vi "Execute.vi"(8 "error in (no error)":errorcluster, 9 "Workspace":T1, 10 "Cluster":T2={"I-O.lvclass"=refnum, "Gantry"=refnum, "Dispenser"="COM1"}, 11 "Pick and Place in":refnum<class "Pick and Place.lvclass">) -> (0 "error out":errorcluster, 2 "Control Out":T2={"I-O.lvclass"=refnum, "Gantry"=refnum, "Dispenser"="COM1"}, 3 "Pick and Place out":refnum<class "Pick and Place.lvclass">)   [LabVIEW 2021, in "Pick and Place.lvclass"]
uses:
  Pick and Place.lvclass
  Controller/Controllers.ctl
  Controller/I-O/I-O.lvclass
  C:/Program Files (x86)/Aerotech/A3200/LabVIEW/2010/Bin/Aerotech.A3200.dll
  Program Files (x86)/Aerotech/A3200/LabVIEW/2010/Bin/Aerotech.A3200.dll
  Workspace/Workspace.ctl
  Pick and Place.lvclass/Pick and Place.ctl
  Controller/Motion/Motion.lvclass
  Controller/Motion/A3200/A3200.lvclass
  Controller/Controller.lvclass
  Workspace/Fixture.lvclass
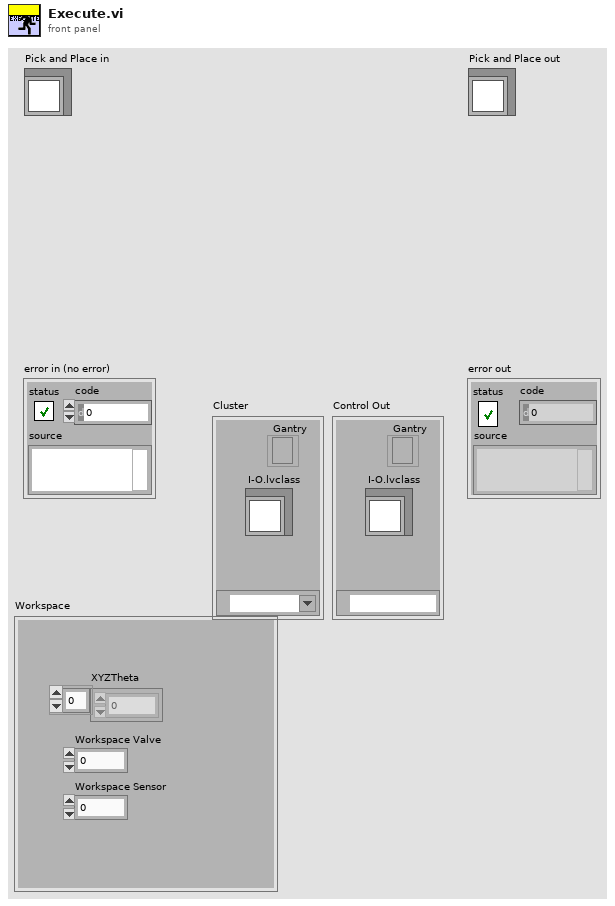
[diagram p1: front panel]
types:
  T1 = typedef "Fixture.lvclass/Workspace.ctl" = cluster{"XYZTheta":dbl[], "Workspace Valve":i32, "Workspace Sensor":i32}
  T2 = typedef "Controller.lvclass/Controllers.ctl" = cluster{"I-O.lvclass":refnum<class "I-O.lvclass">, "Gantry":refnum<k24>, "Dispenser":refnum<visa-resource-name>}
  T3 = typedef "Pick and Place.lvclass/Pick and Place Type.ctl" = enum16{"Primary Pick Up", "Secondary Pick Up", "Put Down All", "Pick Up All", "Put Down Secondary"}
  T4 = typedef "I-O.lvclass/Pin Map.ctl" = cluster{"Region Valves":i32[], "Extra Valves":dbl[][][], "Tool Primary Valve":i32, "Tool Secondary Valve":i32, "Region Sensors":i32[], "Extra Sensors":dbl[][][], "Tool Primary Sensor":dbl, "Tool Secondary Sensor":dbl, "Compression Sensor":dbl, "5V":i32, "Dispenser Sensor":dbl}
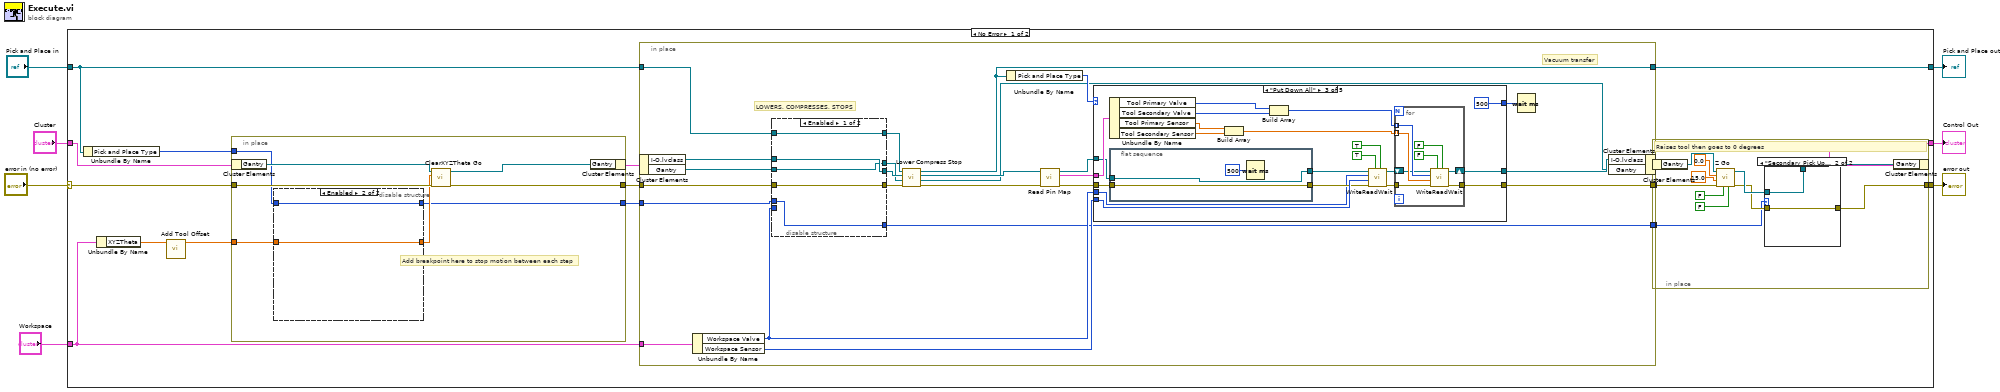
[diagram p0: block diagram]
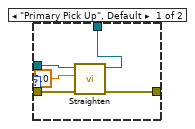
[diagram p2: hidden frame]
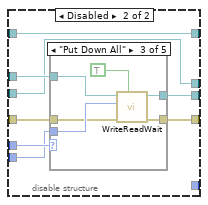
[diagram p3: hidden frame]
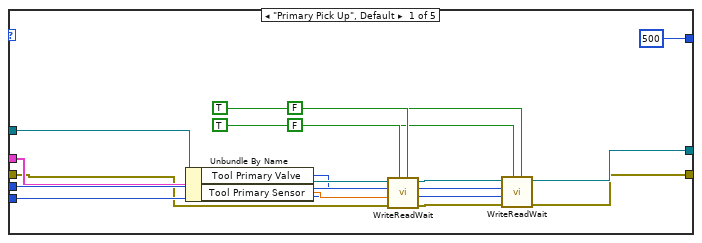
[diagram p8: hidden frame]
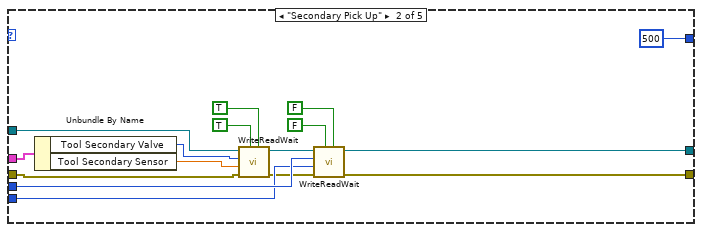
[diagram p9: hidden frame]
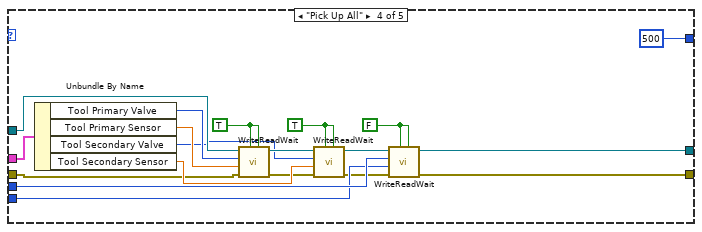
[diagram p10: hidden frame]
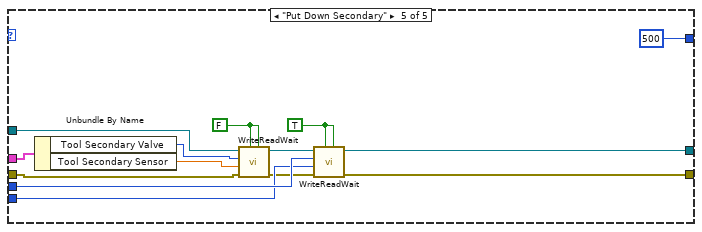
[diagram p11: hidden frame]
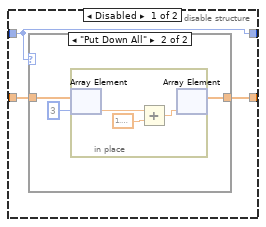
[diagram p12: hidden frame]
diagram:
  n1 = case shown="No Error" "error in (no error)" {
    selector: "error in (no error)" -> [w17 w210]
    tunnel: "Cluster" -> [w21 w211]
    tunnel: "Workspace" -> [w22 _]
    tunnel: [w16 w210] -> w1
    tunnel: [w20 w211] -> w2
    tunnel: "Pick and Place in" -> [w11 w209]
    tunnel: [w19 w209] -> w6
    frame No Error {
      n2 = Unbundle By Name(w11) -> ("Pick and Place Type"=w10:T3)
      n3 = Unbundle By Name(w22) -> ("XYZTheta"=w14:dbl[])
      n4 = call "Add Tool Offset.vi"("XYZTheta"=w14) -> ("Array"=w18:dbl[])  [unwired: 10 in]
      n5 = in-place {
        in-place-border: w18 -> [w191]
        in-place-border: w17 -> [w193]
        in-place-border: [w194] -> w13
        in-place-border: w10 -> [w192]
        in-place-border: [w189] -> w9
        # "Add breakpoint here to stop motion between each step"
        n6 = in-place-cluster #1(w21) -> ("Gantry"=w196:refnum<k24>)
        n7 = disable-structure shown="Enabled" {
          disable-tunnel: w192 -> [w197 w207]
          disable-tunnel: w191 -> [w199 w208]
          disable-tunnel: [w198 w208] -> w190
          disable-tunnel: [w197 w207] -> w189
          frame Disabled {
            n8 = case shown="\"Put Down All\"" w197 {
              tunnel: w199 -> [w200 w203]
              tunnel: [w200 w201] -> w198
              frame "Primary Pick Up", Default {
              }
              frame "Put Down All" {
                n9 = in-place {
                  n10 = in-place-array #2(w203, 3) -> (w206:dbl)
                  n11 = Add(x=w206, y=1.5707963267948966) -> (x+y=w204:dbl)
                  n12 = in-place-array #2(w204) -> (w201:dbl[])  [unwired: 1 out]
                }
              }
            }
          }
          frame Enabled {
          }
        }
        n13 = call "ClearXYZTheta Go.vi"("error in (no error)"=w193, "XYZTheta In"=w190, "Gantry In"=w196) -> ("error out"=w194:errorcluster, "Gantry Out"=w195:refnum<k24>)  [unwired: 6 in, 1 out]
        n14 = in-place-cluster #1("Gantry"=w195) -> (w23:T2)
      }
      n15 = in-place {
        in-place-border: w22 -> [w65]
        in-place-border: w11 -> [w51]
        in-place-border: [w57] -> w19
        in-place-border: w13 -> [w46]
        in-place-border: [w53] -> w12
        in-place-border: w9 -> [w44]
        in-place-border: [w42] -> w8
        # "Vacuum transfer"
        # "LOWERS, COMPRESSES, STOPS"
        n16 = in-place-cluster #3(w23) -> ("I-O.lvclass"=w50:refnum<class "I-O.lvclass">, "Gantry"=w48:refnum<k24>)
        n17 = Unbundle By Name(w65) -> ("Workspace Valve"=w43:i32, "Workspace Sensor"=w63:i32)
        n18 = disable-structure shown="Enabled" {
          disable-tunnel: [w70 w76] -> w52
          disable-tunnel: w51 -> [w70 w76]
          disable-tunnel: w50 -> [w69 w75]
          disable-tunnel: [w69 w74] -> w49
          disable-tunnel: w48 -> [w68 w73]
          disable-tunnel: [w68 w73] -> w47
          disable-tunnel: w46 -> [w67 w72]
          disable-tunnel: [w67 w71] -> w45
          disable-tunnel: w44 -> [w66 w78]
          disable-tunnel: w43 -> [_ w77]
          disable-tunnel: [w66 _] -> w42
          frame Enabled {
          }
          frame Disabled {
            n19 = case shown="\"Put Down All\"" w78 {
              tunnel: w77 -> [_ _ w88 _ _]
              tunnel: w75 -> [w80 w82 w86 w90 w92]
              tunnel: [w80 w82 w85 w90 w92] -> w74
              tunnel: w72 -> [w79 w81 w84 w89 w91]
              tunnel: [w79 w81 w83 w89 w91] -> w71
              frame "Primary Pick Up", Default {
              }
              frame "Secondary Pick Up" {
              }
              frame "Put Down All" {
                n20 = call "WriteReadWait.vi"("Write Value"=TRUE, "error in (no error)"=w84, "Write"=w88, "I-O in"=w86) -> ("error out"=w83:errorcluster, "I-O out"=w85:refnum<class "I-O.lvclass">)  [unwired: 6 in]
              }
              frame "Pick Up All" {
              }
              frame "Put Down Secondary" {
              }
            }
          }
        }
        n21 = call "Lower Compress Stop.vi"("error in (no error)"=w45, "Gantry In"=w47, "I-O.lvclass"=w49, "Pick and Place in"=w52) -> ("error out"=w55:errorcluster, "Gantry Out"=w56:refnum<k24>, "I-O out"=w58:refnum<class "I-O.lvclass">, "Pick and Place Out"=w57:refnum<class "Pick and Place.lvclass">)  [unwired: 4 in]
        n22 = Unbundle By Name(w57) -> ("Pick and Place Type"=w64:T3)
        n23 = call-dynamic "Read Pin Map.vi"("error in (no error)"=w55, "I-O in"=w58) -> ("error out"=w54:errorcluster, "Pin Map 2"=w61:T4, "I-O out"=w60:refnum<class "I-O.lvclass">)  [unwired: 7 in]
        n24 = case shown="\"Put Down All\"" w64 {
          tunnel: w43 -> [w105 w116 w125 w164 w182]
          tunnel: w63 -> [w104 w115 w134 w163 w181]
          tunnel: [w99 w114 w138 w161 w179] -> w59
          tunnel: [u32 500 ("milliseconds to wait") 500 500 u32 500 ("milliseconds to wait") u32 500 ("milliseconds to wait")] -> w62
          tunnel: w60 -> [w98 w113 w130 w173 w187]
          tunnel: w61 -> [w97 w112 w133 w174 w188]
          tunnel: w54 -> [w95 w111 w127 w159 w177]
          tunnel: [w93 w109 w126 w156 w175] -> w53
          frame "Primary Pick Up", Default {
            n25 = Unbundle By Name(w97) -> ("Tool Primary Valve"=w96:i32, "Tool Primary Sensor"=w107:dbl)
            n26 = call "WriteReadWait.vi"("Read Value"=TRUE, "Write Value"=TRUE, "error in (no error)"=w95, "Read"=w107, "Write"=w96, "I-O in"=w98) -> ("error out"=w94:errorcluster, "I-O out"=w106:refnum<class "I-O.lvclass">)  [unwired: 4 in]
            n27 = call "WriteReadWait.vi"("Read Value"=FALSE ("Write Value"), "Write Value"=FALSE ("Read Value"), "error in (no error)"=w94, "Read"=w104, "Write"=w105, "I-O in"=w106) -> ("error out"=w93:errorcluster, "I-O out"=w99:refnum<class "I-O.lvclass">)  [unwired: 4 in]
          }
          frame "Secondary Pick Up" {
            n28 = Unbundle By Name(w112) -> ("Tool Secondary Valve"=w118:i32, "Tool Secondary Sensor"=w117:dbl)
            n29 = call "WriteReadWait.vi"("Read Value"=TRUE, "Write Value"=TRUE, "error in (no error)"=w111, "Read"=w117, "Write"=w118, "I-O in"=w113) -> ("error out"=w110:errorcluster, "I-O out"=w123:refnum<class "I-O.lvclass">)  [unwired: 4 in]
            n30 = call "WriteReadWait.vi"("Read Value"=FALSE ("Write Value"), "Write Value"=FALSE ("Read Value"), "error in (no error)"=w110, "Read"=w115, "Write"=w116, "I-O in"=w123) -> ("error out"=w109:errorcluster, "I-O out"=w114:refnum<class "I-O.lvclass">)  [unwired: 4 in]
          }
          frame "Put Down All" {
            n31 = Unbundle By Name(w133) -> ("Tool Primary Valve"=w139:i32, "Tool Secondary Valve"=w140:i32, "Tool Primary Sensor"=w141:dbl, "Tool Secondary Sensor"=w142:dbl)
            n32 = flat-sequence {
              tunnel: [w146] -> w131
              tunnel: w130 -> [w146]
              tunnel: [w145] -> w128
              tunnel: w127 -> [w145]
              frame #0 {
                # "Delay After Placing"
                n33 = Wait (ms)(milliseconds to wait=u32 500) -> ()  [unwired: 1 out]
              }
            }
            n34 = Build Array(w141, w142) -> (w144:dbl[])
            n35 = Build Array(w139, w140) -> (w143:i32[])
            n36 = call "WriteReadWait.vi"("Read Value"=TRUE, "Write Value"=TRUE, "error in (no error)"=w128, "Read"=w134, "Write"=w125, "I-O in"=w131) -> ("error out"=w129:errorcluster, "I-O out"=w132:refnum<class "I-O.lvclass">)  [unwired: 4 in]
            n37 = for {
              shift-right: [w150] -> w138
              shift-left: w132 -> [w151]
              tunnel: w143 -> [w153] mode=indexing
              tunnel: w144 -> [w152] mode=indexing
              tunnel: w129 -> [w149]
              tunnel: [w148] -> w126
              n38 = call "WriteReadWait.vi"("Read Value"=FALSE ("Write Value"), "Write Value"=FALSE ("Read Value"), "error in (no error)"=w149, "Read"=w152, "Write"=w153, "I-O in"=w151) -> ("error out"=w148:errorcluster, "I-O out"=w150:refnum<class "I-O.lvclass">)  [unwired: 4 in]
            }
          }
          frame "Pick Up All" {
            w162 = FALSE ("Read Value")
            w166 = TRUE ("Write Value")
            w172 = TRUE ("Write Value")
            n39 = Unbundle By Name(w174) -> ("Tool Primary Valve"=w171:i32, "Tool Primary Sensor"=w170:dbl, "Tool Secondary Valve"=w168:i32, "Tool Secondary Sensor"=w167:dbl)
            n40 = call "WriteReadWait.vi"("Read Value"=w172, "Write Value"=w172, "error in (no error)"=w159, "Read"=w170, "Write"=w171, "I-O in"=w173) -> ("error out"=w158:errorcluster, "I-O out"=w169:refnum<class "I-O.lvclass">)  [unwired: 4 in]
            n41 = call "WriteReadWait.vi"("Read Value"=w166, "Write Value"=w166, "error in (no error)"=w158, "Read"=w167, "Write"=w168, "I-O in"=w169) -> ("error out"=w157:errorcluster, "I-O out"=w165:refnum<class "I-O.lvclass">)  [unwired: 4 in]
            n42 = call "WriteReadWait.vi"("Read Value"=w162, "Write Value"=w162, "error in (no error)"=w157, "Read"=w163, "Write"=w164, "I-O in"=w165) -> ("error out"=w156:errorcluster, "I-O out"=w161:refnum<class "I-O.lvclass">)  [unwired: 4 in]
          }
          frame "Put Down Secondary" {
            w180 = TRUE ("Read Value")
            w184 = FALSE ("Write Value")
            n43 = Unbundle By Name(w188) -> ("Tool Secondary Valve"=w186:i32, "Tool Secondary Sensor"=w185:dbl)
            n44 = call "WriteReadWait.vi"("Read Value"=w184, "Write Value"=w184, "error in (no error)"=w177, "Read"=w185, "Write"=w186, "I-O in"=w187) -> ("error out"=w176:errorcluster, "I-O out"=w183:refnum<class "I-O.lvclass">)  [unwired: 4 in]
            n45 = call "WriteReadWait.vi"("Read Value"=w180, "Write Value"=w180, "error in (no error)"=w176, "Read"=w181, "Write"=w182, "I-O in"=w183) -> ("error out"=w175:errorcluster, "I-O out"=w179:refnum<class "I-O.lvclass">)  [unwired: 4 in]
          }
        }
        n46 = Wait (ms)(milliseconds to wait=w62) -> ()  [unwired: 1 out]
        n47 = in-place-cluster #3("I-O.lvclass"=w59, "Gantry"=w56) -> (w15:T2)
      }
      n48 = in-place {
        in-place-border: [w26] -> w16
        in-place-border: w12 -> [w32]
        in-place-border: w8 -> [w24]
        # "Raises tool then goes to 0 degrees"
        n49 = in-place-cluster #4(w15) -> ("Gantry"=w29:refnum<k24>)
        n50 = call "Z Go.vi"("Increment"=FALSE, "Return Immediately"=FALSE ("Increment"), "error in (no error)"=w32, "Speed In"=15.0 ("speed"), "Position In"=0.0 ("position"), "Gantry In"=w29) -> ("error out"=w27:errorcluster, "Gantry Out"=w31:refnum<k24>)  [unwired: 2 in, 2 out]
        n51 = case shown="\"Secondary Pick Up\"" w24 {
          tunnel: w31 -> [w39 w40]
          tunnel: [w38 w40] -> w30
          tunnel: w27 -> [w37 w41]
          tunnel: [w36 w41] -> w26
          frame "Primary Pick Up", Default {
            n52 = call "Straighten.vi"("error in (no error)"=w37, "Angle (rad)"=0.0, "Gantry In"=w39) -> ("error out"=w36:errorcluster, "Gantry Out"=w38:refnum<k24>)  [unwired: 7 in]
          }
          frame "Secondary Pick Up" {
          }
        }
        n53 = in-place-cluster #4("Gantry"=w30) -> (w20:T2)
      }
    }
    frame Error {
    }
  }
  "error out" <- w1
  "Pick and Place out" <- w6
  "Control Out" <- w2
